vi "CustomCommandSubVI.vi"(3 "Send_command":bool, 4 "Command":string, 5 "TCP Network Connection in":refnum<k5>) -> (0 "error out":errorcluster, 1 "bytes written":i32, 2 "TCP Network Connection out":refnum<k5>)   [LabVIEW 2020]
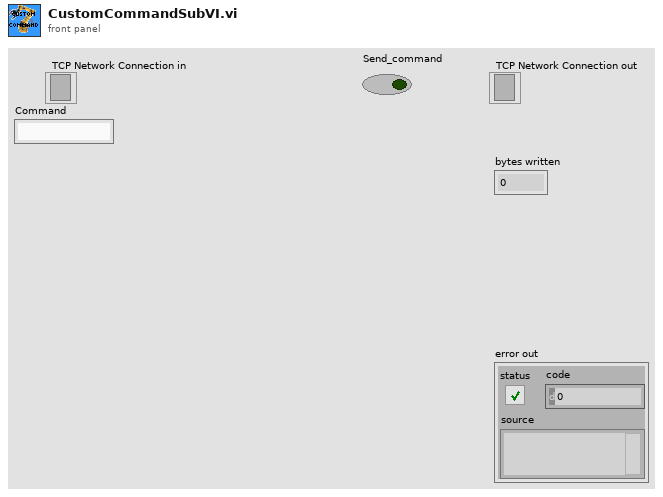
[diagram p1: front panel]
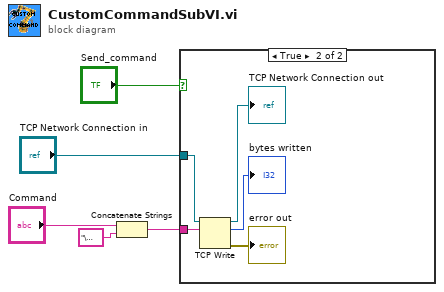
[diagram p0: block diagram]
diagram:
  n1 = Concatenate Strings("Command", "\u0000") -> (w1:string)
  n2 = case shown="True" "Send_command" {
    tunnel: "TCP Network Connection in" -> [_ w10]
    tunnel: w1 -> [_ w6]
    frame False {
    }
    frame True {
      n3 = TCP Write(connection ID=w10, data in=w6) -> (connection ID out=→"TCP Network Connection out":refnum<k5>, bytes written=→"bytes written":i32, error out=→"error out":errorcluster)  [unwired: 2 in]
    }
  }
